vi "Memory Throughput Test PXI-795XR (Host).vi"() -> ()   [LabVIEW 2013]
doc: "This example writes to and reads from external memory at various data rates and reports the total measured throughput. Varying the write and read grant time directly affects the memory efficiency. The larger the grant time, then the larger the throughput, and the lower the grant time, then the lower the throughput.\n\nDuring reads, the data is validated against an expected pattern. Failures will cause \"Read Data Error?\" to illuminate. To avoid read data errors, a full iteration of memory writes must be completed before starting the memory reads."
uses:
  <vilib>/FPGAPlugInAG/PXI-7954R/niLvFpga_Open_PXI-7954R.vi
  <vilib>/FPGAPlugInAG/PXI-7954R/niLvFpga_Download_PXI-7954R.vi
  <vilib>/FPGAPlugInAG/PXI-7954R/niLvFpga_Reset_PXI-7954R.vi
  <vilib>/Utility/error.llb/Error Cluster From Error Code.vi
  <vilib>/rvi/errors/niLvFpgaAdjustHostInterfaceError.vi
  <vilib>/FPGAPlugInAG/PXI-7954R/niLvFpga_Run_PXI-7954R.vi
  <vilib>/FPGAPlugInAG/PXI-7954R/niLvFpga_Close_PXI-7954R.vi
  <vilib>/rvi/interface/nirviOpenFPGA/nirviOpenFPGA.xnode
  Program Files (x86)/National Instruments/LabVIEW 2013/examples/FlexRIO/External Memory/Memory Throughput Test/FPGA Bitfiles/MemoryThro_PXI-7954R.lvbitx
  Program Files (x86)/National Instruments/LabVIEW 2013/examples/FlexRIO/External Memory/Memory Throughput Test/Memory Throughput Test PXI-795XR (FPGA).vi
  <vilib>/rvi/interface/nirviMethod/nirviMethod.xnode
  <vilib>/rvi/interface/nirviReadWriteControl/nirviReadWriteControl.xnode
  <vilib>/rvi/interface/nirviCloseFPGA/nirviCloseFPGA.xnode
  NiFpgaLv.dll
panel:
  in  "Read Req Grant Time (Bank 1)":u16=1000 caption="Read Req Grant Time (clocks)"
  in  "Write Req Grant Time (Bank 1)":u16=1000 caption="Write Req Grant Time (clocks)"
  out "Read FIFO Overflow? (Bank 0)":bool caption="Read FIFO Overflow?"
  in  "Read Req Grant Time (Bank 0)":u16=1000 caption="Read Req Grant Time (clocks)"
  in  "Write Req Grant Time (Bank 0)":u16=1000 caption="Write Req Grant Time  (clocks)"
  out "Read Data Error? (Bank 1)":bool caption="Read Data Error?"
  out "Read FIFO Overflow? (Bank 1)":bool caption="Read FIFO Overflow?"
  out "Read Data Error? (Bank 0)":bool caption="Read Data Error?"
  out "Current Read Data (Bank 1)":u64 caption="Current Read Data" format="%.0x"
  out "Read Throughput (bytes/sec) (Bank 1)":u32 caption="Read Throughput (bytes/sec)" format="%^.1e"
  out "Read Throughput (bytes/sec) (Bank 0)":u32 caption="Read Throughput (bytes/sec)" format="%^.1e"
  out "Current Read Data (Bank 0)":u64 caption="Current Read Data" format="%.0x"
  out "Current Read Address (Bank 1)":u32 caption="Current Read Address" format="%.0x"
  in  "Enable Reads? (Bank 1)":bool caption="Enable Reads?"
  in  "Enable Reads? (Bank 0)":bool caption="Enable Reads?"
  out "Current Read Address (Bank 0)":u32 caption="Current Read Address" format="%.0x"
  out "Current Write Data (Bank 1)":u64 caption="Current Write Data" format="%.0x"
  out "Current Write Address (Bank 1)":u32 caption="Current Write Address" format="%.0x"
  in  "Enable Writes? (Bank 1)":bool=TRUE caption="Enable Writes?"
  out "Write Throughput (bytes/sec) (Bank 1)":u32 caption="Write Throughput (bytes/sec)" format="%^.1e"
  in  "DRAM Size (elements) (Bank 1)":u32=8388608 caption="DRAM Size (elements)"
  out "Write Throughput (bytes/sec) (Bank 0)":u32 caption="Write Throughput (bytes/sec)" format="%^.1e"
  in  "Enable Writes? (Bank 0)":bool=TRUE caption="Enable Writes?"
  out "Current Write Data (Bank 0)":u64 caption="Current Write Data" format="%.0x"
  in  "DRAM Size (elements) (Bank 0)":u32=8388608 caption="DRAM Size (elements)"
  out "Current Write Address (Bank 0)":u32 caption="Current Write Address" format="%.0x"
  in  "stop":bool
  # "Bank 0"
  # "Bank 1"
  # "This test writes to and reads from external memory at maximum data rates and reports the total measured throughput.  Varying the write and read grant time will directly affect the memory efficiency.  The larger the grant time, then the larger the througput, and the lower the grant time, then the lower the throughput \n\nDuring reads, the data is validated against an expected pattern.  Failures will cause \"Read Data Error?\" to illuminate.  To avoid read data errors, a full iteration of memory writes must be completed before starting the memory reads."
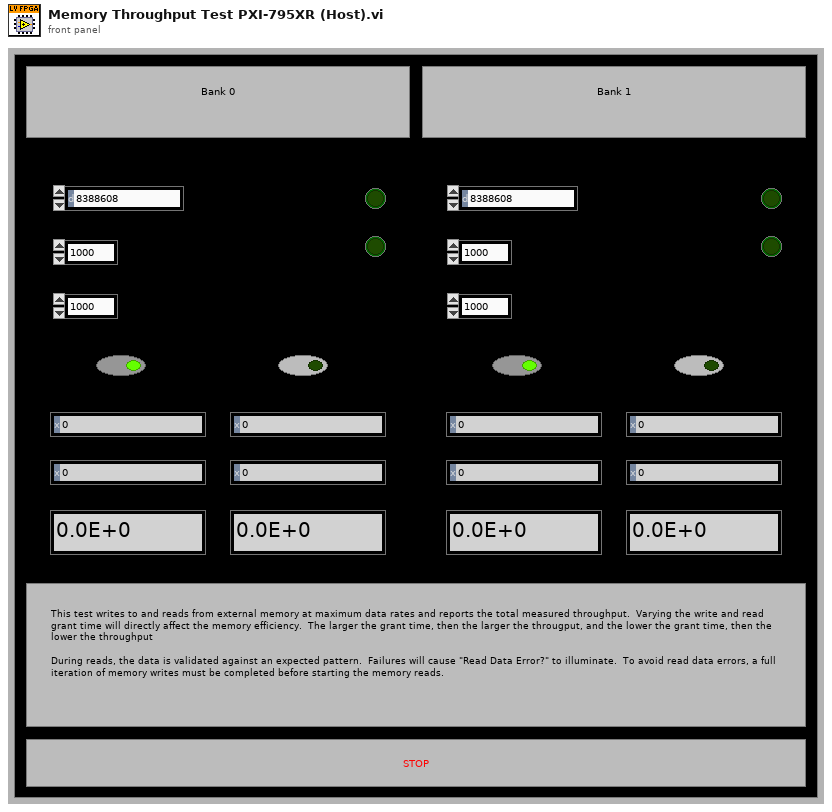
[diagram p1: front panel]
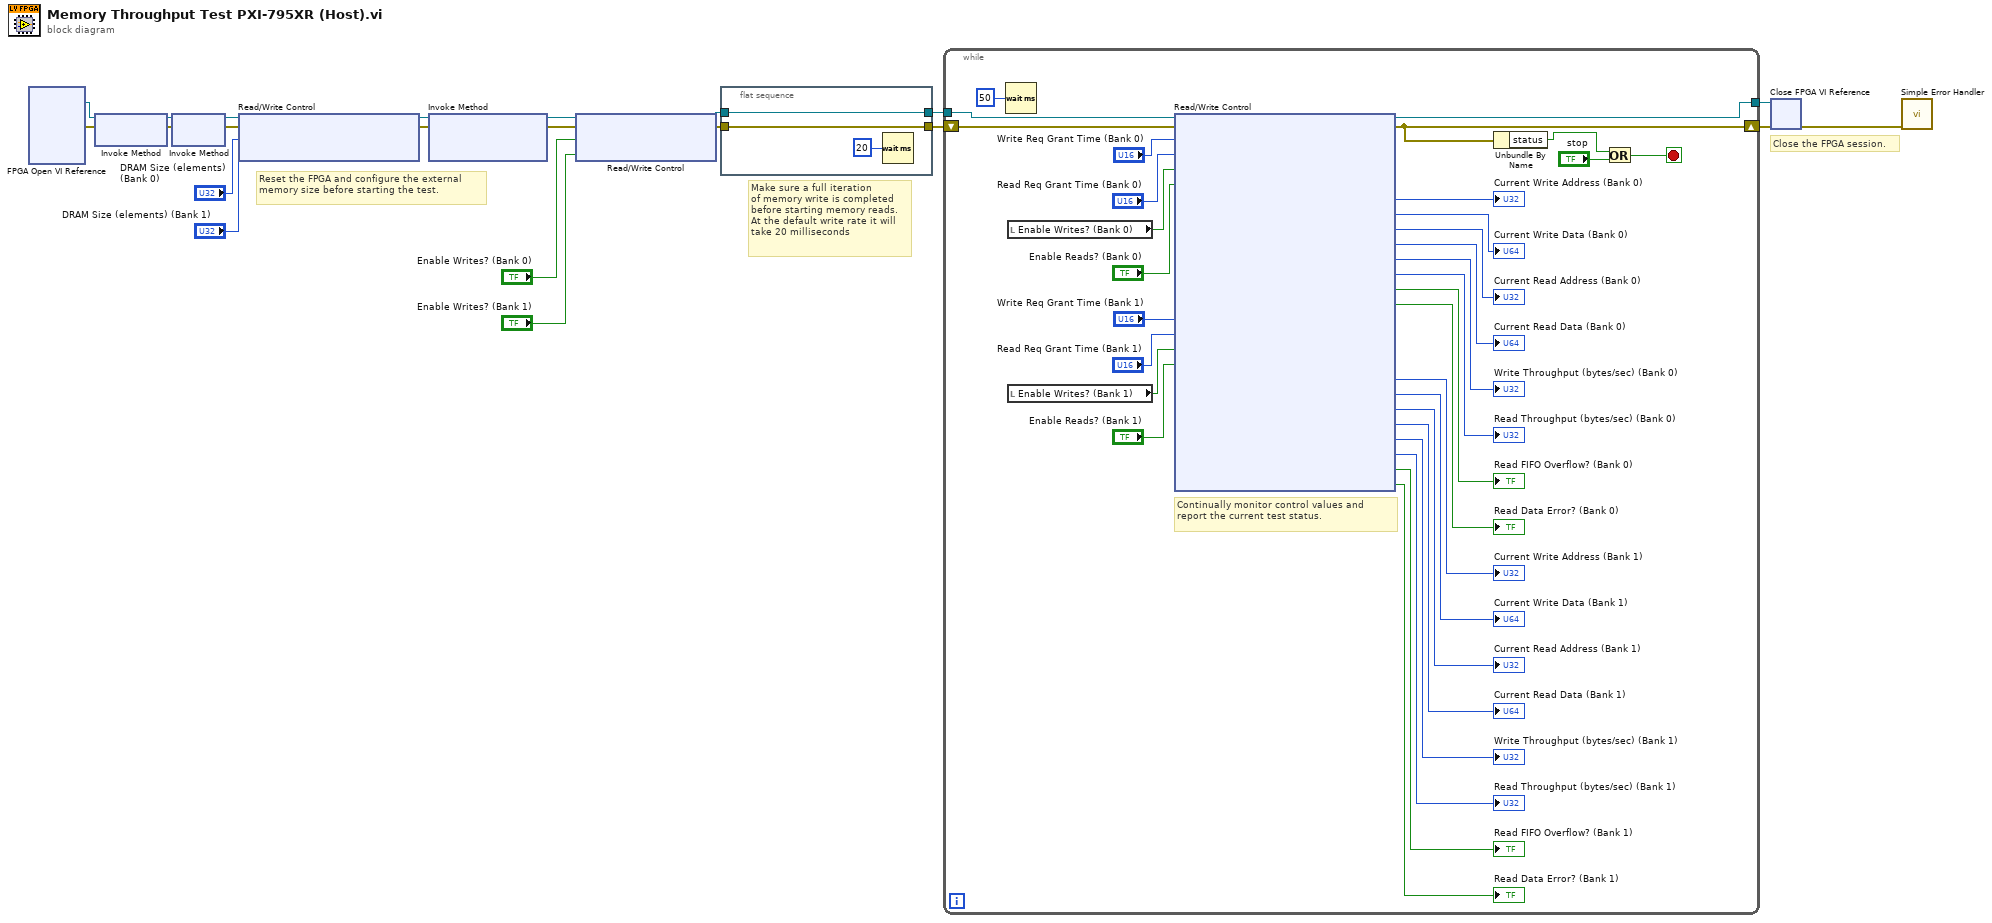
[diagram p0: block diagram]
diagram:
  # "Make sure a full iteration\nof memory write is completed\nbefore starting memory reads.\nAt the default write rate it will \ntake 20 milliseconds"
  # "Close the FPGA session."
  # "Reset the FPGA and configure the external memory size before starting the test."
  n1 = xnode "FPGA Open VI Reference"() -> ("FPGA VI Reference Out"=w16:refnum<k20>, "error out"=w17:errorcluster)  [unwired: 2 in]
  n2 = xnode "Invoke Method"("FPGA VI Reference In"=w16, "error in"=w17) -> ("FPGA VI Reference Out"=w3:refnum<k20>, "error out"=w4:errorcluster)
  n3 = xnode "Invoke Method"("FPGA VI Reference In"=w3, "error in"=w4) -> ("FPGA VI Reference Out"=w6:refnum<k20>, "error out"=w5:errorcluster)
  n4 = xnode "Read/Write Control"("FPGA VI Reference In"=w6, "error in"=w5, "DRAM Size (elements) (Bank 0)"="DRAM Size (elements) (Bank 0)", "DRAM Size (elements) (Bank 1)"="DRAM Size (elements) (Bank 1)") -> ("FPGA VI Reference Out"=w20:refnum<k20>, "error out"=w21:errorcluster)
  n5 = xnode "Invoke Method"("FPGA VI Reference In"=w20, "error in"=w21) -> ("FPGA VI Reference Out"=w11:refnum<k20>, "error out"=w12:errorcluster)  [unwired: 1 in]
  n6 = xnode "Read/Write Control"("FPGA VI Reference In"=w11, "error in"=w12, "Enable Writes? (Bank 0)"="Enable Writes? (Bank 0)", "Enable Writes? (Bank 1)"="Enable Writes? (Bank 1)") -> ("FPGA VI Reference Out"=w10:refnum<k20>, "error out"=w8:errorcluster)
  n7 = flat-sequence {
    tunnel: w10 -> [w24]
    tunnel: [w24] -> w9
    tunnel: w8 -> [w23]
    tunnel: [w23] -> w7
    frame #0 {
      n8 = Wait (ms)(milliseconds to wait=u32 20) -> ()  [unwired: 1 out]
    }
  }
  n9 = while {
    shift-right: [w51] -> w19
    shift-left: w7 -> [w49]
    tunnel: w9 -> [w50]
    tunnel: [w52] -> w15
    stop <- w56 stop-if-true
    # "Continually monitor control values and report the current test status."
    n10 = Wait (ms)(milliseconds to wait=u32 50) -> ()  [unwired: 1 out]
    n11 = local read "Enable Writes? (Bank 0)"() -> (w48:bool)
    n12 = local read "Enable Writes? (Bank 1)"() -> (w46:bool)
    n13 = xnode "Read/Write Control"("FPGA VI Reference In"=w50, "error in"=w49, "Write Req Grant Time (Bank 0)"="Write Req Grant Time (Bank 0)", "Read Req Grant Time (Bank 0)"="Read Req Grant Time (Bank 0)", "Enable Writes? (Bank 0)"=w48, "Enable Reads? (Bank 0)"="Enable Reads? (Bank 0)", "Write Req Grant Time (Bank 1)"="Write Req Grant Time (Bank 1)", "Read Req Grant Time (Bank 1)"="Read Req Grant Time (Bank 1)", "Enable Writes? (Bank 1)"=w46, "Enable Reads? (Bank 1)"="Enable Reads? (Bank 1)") -> ("FPGA VI Reference Out"=w52:refnum<k20>, "error out"=w51:errorcluster, "Current Write Address (Bank 0)"=→"Current Write Address (Bank 0)":u32, "Current Write Data (Bank 0)"=→"Current Write Data (Bank 0)":u64, "Current Read Address (Bank 0)"=→"Current Read Address (Bank 0)":u32, "Current Read Data (Bank 0)"=→"Current Read Data (Bank 0)":u64, "Write Throughput (bytes/sec) (Bank 0)"=→"Write Throughput (bytes/sec) (Bank 0)":u32, "Read Throughput (bytes/sec) (Bank 0)"=→"Read Throughput (bytes/sec) (Bank 0)":u32, "Read FIFO Overflow? (Bank 0)"=→"Read FIFO Overflow? (Bank 0)":bool, "Read Data Error? (Bank 0)"=→"Read Data Error? (Bank 0)":bool, "Current Write Address (Bank 1)"=→"Current Write Address (Bank 1)":u32, "Current Write Data (Bank 1)"=→"Current Write Data (Bank 1)":u64, "Current Read Address (Bank 1)"=→"Current Read Address (Bank 1)":u32, "Current Read Data (Bank 1)"=→"Current Read Data (Bank 1)":u64, "Write Throughput (bytes/sec) (Bank 1)"=→"Write Throughput (bytes/sec) (Bank 1)":u32, "Read Throughput (bytes/sec) (Bank 1)"=→"Read Throughput (bytes/sec) (Bank 1)":u32, "Read FIFO Overflow? (Bank 1)"=→"Read FIFO Overflow? (Bank 1)":bool, "Read Data Error? (Bank 1)"=→"Read Data Error? (Bank 1)":bool)
    n14 = Unbundle By Name(w51) -> ("status"=w54:bool)
    n15 = Or(x=w54, y="stop") -> (x .or. y?=w56:bool)
  }
  n16 = xnode "Close FPGA VI Reference"("FPGA VI Reference In"=w15, "error in"=w19) -> ("error out"=w18:errorcluster)
  n17 = call <vilib>:"Simple Error Handler.vi"("error in (no error)"=w18) -> ()  [unwired: 1 in, 8 out]
